vi "Day 16-Parse Input.vi"(11 "String in":string) -> (3 "String out":string)   [LabVIEW 2021]
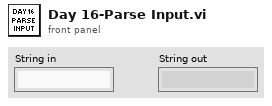
[diagram p1: front panel]
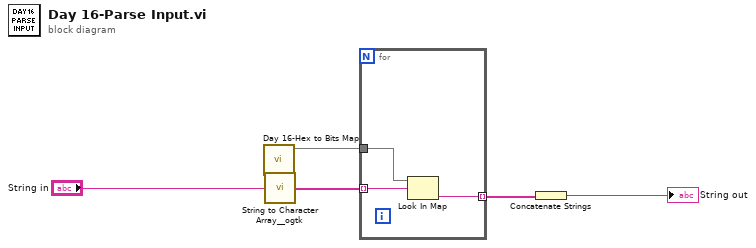
[diagram p0: block diagram]
diagram:
  n1 = call "Day 16-Hex to Bits Map.vi"() -> ("Map"=w3:map{string, string})  [unwired: 11 in]
  n2 = call <userlib>:"String to Character Array__ogtk.vi"("Input String"="String in") -> ("Character Array"=w2:string[])
  n3 = for {
    tunnel: w2 -> [w7] mode=indexing
    tunnel: w3 -> [w8]
    tunnel: [w6] -> w4 mode=indexing
    n4 = Look In Map(map=w8, key=w7) -> (value=w6:string)  [unwired: 1 in, 1 out]
  }
  n5 = Concatenate Strings(w4) -> (→"String out":string)
